vi "Setup subWorkers.vi"(8 "error in":errorcluster, 11 "Network End Point in":refnum<class "Network End Point.lvclass">) -> (0 "error out":errorcluster, 3 "Network End Point out":refnum<class "Network End Point.lvclass">)   [LabVIEW 2020, in "Network End Point.lvclass"]
doc: "<b>Note: Do not change the code in this VI!</b>\nThis VI performs a setup of all the statically-linked subWorkers that belong to the Worker that calls this VI. This VI is created automatically by the 'Create/Add Worker' tool and must be called <b>before</b> any statically linked subWorkers are called."
uses:
  Network End Point.lvclass
  C:/Program Files (x86)/National Instruments/LabVIEW 2020/vi.lib/addons/_Workers/Library/Classes/Worker/Worker.lvclass
  subWorkers.ctl
  TCP Send/TCP Send.lvclass
  TCP Receive/TCP Receive.lvclass
  Network End Point.lvclass/Network End Point.ctl
  <vilib>/addons/_Workers/Library/Classes/Worker/Worker.lvclass
panel:
  out "subWorkers":T1
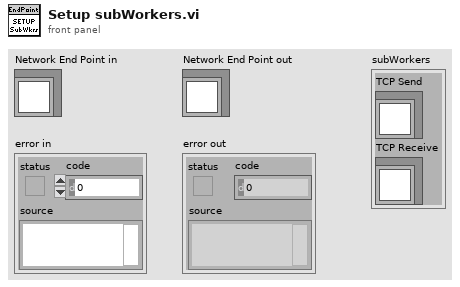
[diagram p1: front panel]
types:
  T1 = typedef "Network End Point.lvclass/subWorkers.ctl" = cluster{"TCP Send":refnum<class "TCP Send.lvclass">, "TCP Receive":refnum<class "TCP Receive.lvclass">}
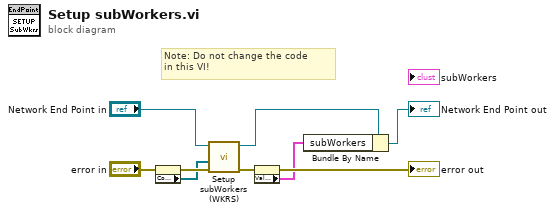
[diagram p0: block diagram]
diagram:
  # "Note: Do not change the code \nin this VI!"
  n1 = property on="subWorkers" class="Clust (strict)"(error in="error in") -> (error out=w7:errorcluster, "Controls[]"=w4:refnum<vi>[])  [unwired: 1 in, 1 out]
  n2 = call <vilib>:"Setup subWorkers (WKRS).vi"("error in"=w7, "Controls[]"=w4, "Worker"="Network End Point in") -> ("error out"=w5:errorcluster, "Worker out"=w1:refnum<class "Network End Point.lvclass">)  [unwired: 7 in]
  n3 = property on="subWorkers" class="Clust (strict)"(error in=w5) -> (error out=→"error out":errorcluster, "Value"=w3:T1)  [unwired: 1 in, 1 out]
  n4 = Bundle By Name(cluster=w1, "subWorkers"=w3) -> (→"Network End Point out":refnum<class "Network End Point.lvclass">)
